vi "Teleop.vi"(1 "PreValue 2":bool, 3 "PreValue":bool, 9 "PreValue 3":bool, 10 "Match Info":T1={"Autonomous Elapsed Seconds"=0.0, "TeleOp Elapsed Seconds"=0.0, "Disabled Elapsed Seconds"=0.0, "Visited Autonomous"=FALSE, "Visited TeleOp"=FALSE, "Visited Disabled"=FALSE, "Autonomous Settings"={"Autonomous Style"=enum."Independent", "VI Refnum"=refnum}}, 11 "Call Context":T2) -> (0 "CurrentValue 2":bool, 2 "CurrentValue":bool, 8 "CurrentValue 3":bool)   [LabVIEW 2015]
doc: "This VI is called for each TeleOp packet received from the DS where the robot is not disabled. It is often used to read from the joysticks and update I/O or to update setpoints for timed control loops. It should complete and return within 20 milliseconds or it may miss DS packets."
uses:
  <vilib>/Rock Robotics/WPI/DriverStation/WPI_DriverStationDerivedRobotMode.ctl
  <vilib>/Rock Robotics/WPI/DriverStation/WPI_DriverStationMatch Info.ctl
  <vilib>/Rock Robotics/WPI/Solenoid/WPI_SolenoidValue.ctl
  <vilib>/Rock Robotics/WPI/Utilities/WPI_GetSetVariantRefNum.vi
  <vilib>/Rock Robotics/Network Tables/NT Write Boolean.vi
  <vilib>/Rock Robotics/Network Tables/NT Write Numeric Array.vi
  <vilib>/Rock Robotics/Network Tables/NT Read Boolean.vi
  <vilib>/Rock Robotics/Network Tables/NT Read Number.vi
  Robot Global Data.vi
  <vilib>/Rock Robotics/WPI/Solenoid/WPI_SolenoidSetEnum.vi
panel:
  out "Sample Slider 0":dbl(slide) scale=0.0..5.0
  out "Sample Boolean 1":bool
  out "Sample Boolean 0":bool
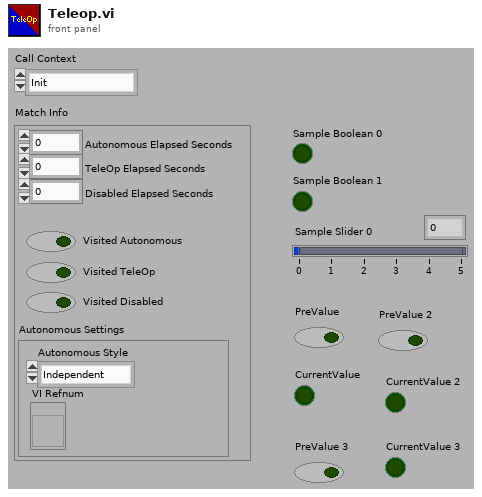
[diagram p1: front panel]
types:
  T1 = typedef "WPI_DriverStationMatch Info.ctl" = cluster{"Autonomous Elapsed Seconds":dbl, "TeleOp Elapsed Seconds":dbl, "Disabled Elapsed Seconds":dbl, "Visited Autonomous":bool, "Visited TeleOp":bool, "Visited Disabled":bool, "Autonomous Settings":cluster{"Autonomous Style":enum16{"Iterative", "Independent"}, "VI Refnum":refnum<vi>}}
  T2 = typedef "WPI_DriverStationDerivedRobotMode.ctl" = enum16{"Init", "Execute", "Stop"}
  T3 = typedef "WPI_SolenoidValue.ctl" = enum16{"Off", "On", "Forward", "Reverse"}
  T4 = typedef "WPI_RobotDriveDevRef.ctl" = cluster{"DevStatus":errorcluster, "Motors[]":T5[], "Square Inputs":bool, "Max Output":dbl}
  T5 = typedef "WPI_MotorControlDeviceRef.ctl" = cluster{"DeviceStatus":errorcluster, "Type":T6, "PWM":cluster{"PWM Channel":T7, "DeadBand":T8}, "CAN":cluster{"Device Number":u8, "Control Mode":T9, "Semaphore":T10, "Max Vout":dbl, "TalonSRX Control Mode":T11}, "Invert":bool}
  T6 = typedef "WPI_MotorControlType.ctl" = enum16{"PWM", "CAN", "CANTalonSRX"}
  T7 = typedef "FPGA_DIOPWMChannel.ctl" = enum8{"PWM 0", "PWM 1", "PWM 2", "PWM 3", "PWM 4", "PWM 5", "PWM 6", "PWM 7", "PWM 8", "PWM 9", "PWM MXP 0", "PWM MXP 1", "PWM MXP 2", "PWM MXP 3", "PWM MXP 4", "PWM MXP 5", "PWM MXP 6", "PWM MXP 7", "PWM MXP 8", "PWM MXP 9", "Invalid"}
  T8 = typedef "WPI_PWMDeadband.ctl" = cluster{"Name":string, "maxPositivePwm":i32, "minPositivePwm":i32, "centerPwm":i32, "maxNegativePwm":i32, "minNegativePwm":i32, "angularRange":u16}
  T9 = typedef "WPI_CANJaguar_ControlMode.ctl" = enum8{"Percent VBus", "Current", "Speed", "Position", "Voltage"}
  T10 = typedef "Semaphore RefNum" = refnum<k1>
  T11 = typedef "WPI_CANTalonSRX_APIControlMode.ctl" = enum8{"Percent VBus", "Speed", "Position", "Slave", "Unchanged / Invalid", "Voltage Compensation", "Current", "Motion Profile"}
  T12 = typedef "WPI_JoystickDevRef.ctl" = cluster{"Device":T13}
  T13 = typedef "WPI_JoystickDeviceEnum.ctl" = enum16{"USB 0", "USB 1", "USB 2", "USB 3", "USB 4", "USB 5"}
  T14 = cluster{"Buttons[0]":bool, "Buttons[1]":bool, "Buttons[2]":bool, "Buttons[3]":bool, "Buttons[4]":bool, "Buttons[5]":bool, "Buttons[6]":bool, "Buttons[7]":bool, "Buttons[8]":bool}
  T15 = typedef "WPI_DigitalInputDevRef.ctl" = cluster{"DevStatus":errorcluster, "DIO Channel":T16}
  T16 = typedef "FPGA_DIOChannel.ctl" = enum8{"DIO 0", "DIO 1", "DIO 2", "DIO 3", "DIO 4", "DIO 5", "DIO 6", "DIO 7", "DIO 8", "DIO 9", "DIO MXP 0", "DIO MXP 1", "DIO MXP 2", "DIO MXP 3", "DIO MXP 4", "DIO MXP 5", "DIO MXP 6", "DIO MXP 7", "DIO MXP 8", "DIO MXP 9", "DIO MXP 10", "DIO MXP 11", "DIO MXP 12", "DIO MXP 13", "DIO MXP 14", "DIO MXP 15", "Invalid"}
  T17 = typedef "WPI_SolenoidDevRef.ctl" = cluster{"DevStatus":errorcluster, "Pneumatics Control Module":u8, "Forward Solenoid Channel":T18, "Reverse Solenoid Channel":T18}
  T18 = typedef "WPI_SolenoidChannel.ctl" = enum8{"Solenoid 0", "Solenoid 1", "Solenoid 2", "Solenoid 3", "Solenoid 4", "Solenoid 5", "Solenoid 6", "Solenoid 7", "Invalid"}
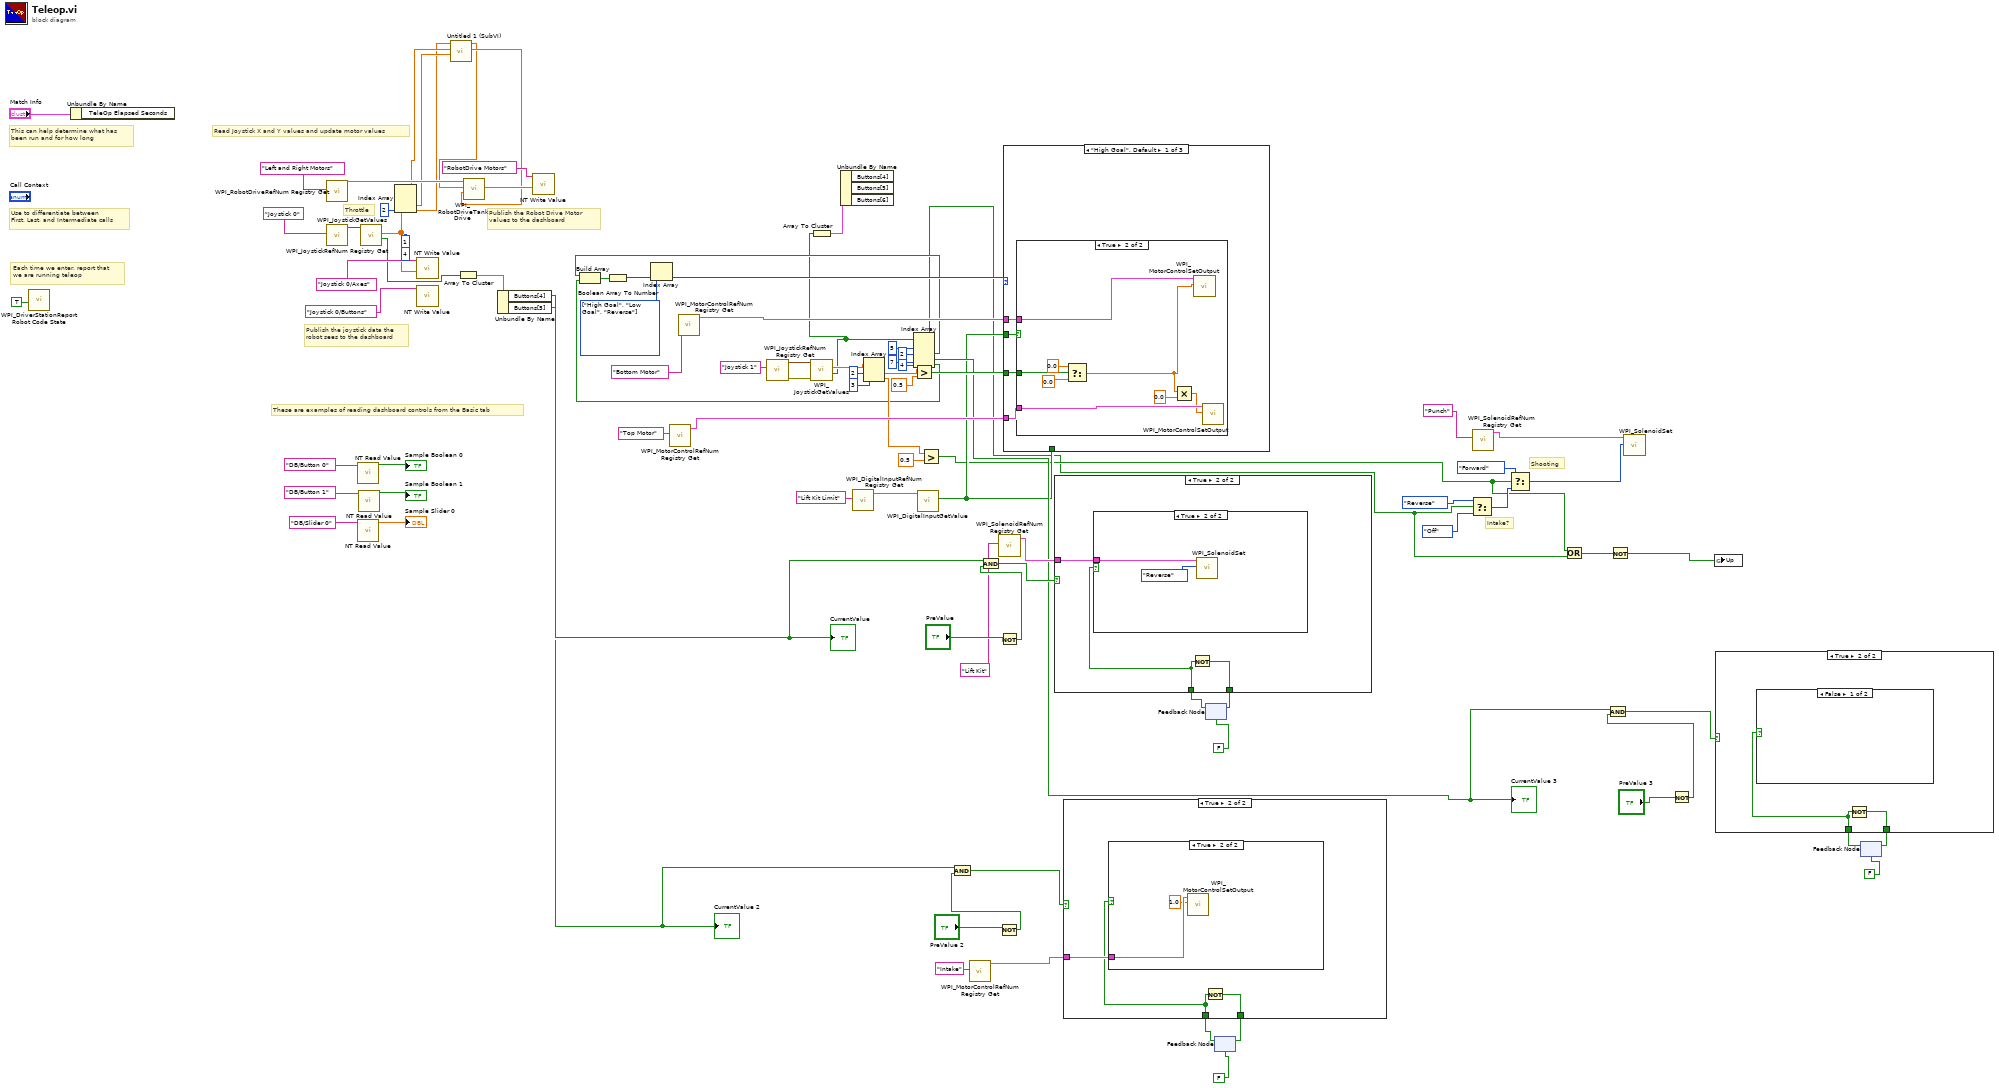
[diagram p0: block diagram]
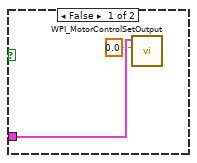
[diagram p5: hidden frame]
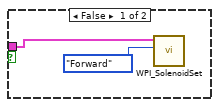
[diagram p7: hidden frame]
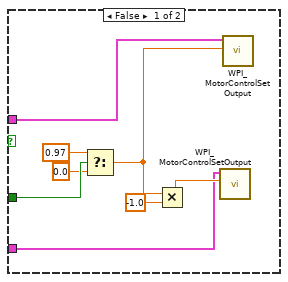
[diagram p8: hidden frame]
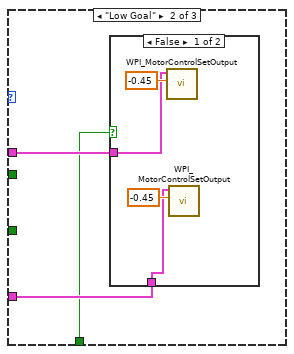
[diagram p9: hidden frame]
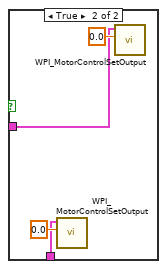
[diagram p10: hidden frame]
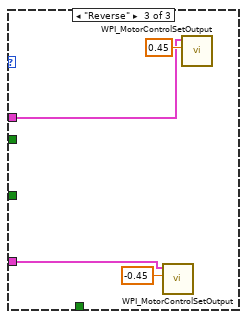
[diagram p11: hidden frame]
diagram:
  w75 = enum16{"High Goal", "Low Goal", "Reverse", ""}[] [enum."High Goal", enum."Low Goal", enum."Reverse"] items=["High Goal", "Low Goal", "Reverse", ""] ("array")
  # "Throttle"
  # "Intake?"
  # "Shooting"
  # "These are examples of reading dashboard controls from the Basic tab"
  # "Publish the Robot Drive Motor\nvalues to the dashboard"
  # "Publish the joystick data the\nrobot sees to the dashboard"
  # "Each time we enter, report that\nwe are running teleop"
  # "Use to differentiate between\nFirst, Last, and Intermediate calls"
  # "This can help determine what has\nbeen run and for how long"
  # "Read Joystick X and Y values and update motor values"
  n1 = call <vilib>:"WPI_DriverStationReport Robot Code State.vi"("TeleOp"=TRUE ("Autonomous")) -> ()  [unwired: 10 in, 1 out]
  n2 = Unbundle By Name("Match Info") -> ()  [unwired: 1 out]
  n3 = call <vilib>:"WPI_RobotDriveRefNum Registry Get.vi"("refnum name"="Left and Right Motors") -> ("RobotDriveDevRef"=w58:T4)  [unwired: 1 in, 9 out]
  n4 = call <vilib>:"WPI_JoystickRefNum Registry Get.vi"("refnum name"="Joystick 0") -> ("JoystickDevRef"=w90:T12)  [unwired: 1 in, 9 out]
  n5 = call-poly <vilib>:"NT Read Value.vi"("Name"="DB/Button 0" ("refnum name")) -> ("Boolean"=→"Sample Boolean 0":bool)  [unwired: 9 in, 1 out]
  n6 = call-poly <vilib>:"NT Read Value.vi"("Name"="DB/Slider 0" ("refnum name")) -> ("Numeric"=→"Sample Slider 0":dbl)  [unwired: 9 in, 1 out]
  n7 = call-poly <vilib>:"NT Read Value.vi"("Name"="DB/Button 1" ("refnum name")) -> ("Boolean"=→"Sample Boolean 1":bool)  [unwired: 9 in, 1 out]
  n8 = call <vilib>:"WPI_JoystickGetValues.vi"("JoystickDevRef"=w90) -> ("Buttons"=w71:bool[], "Axes"=w86:dbl[])  [unwired: 6 in, 3 out]
  n9 = Index Array(array=w86, index #1=1 ("index"), index #2=4 ("index"), index #3=2 ("index")) -> (element #1=w28:dbl, element #2=w29:dbl, element #3=w24:dbl)
  n10 = call-poly <vilib>:"NT Write Value.vi"("Numeric Array"=w86, "Name"="Joystick 0/Axes") -> ()  [unwired: 9 in, 1 out]
  n11 = call-poly <vilib>:"NT Write Value.vi"("Name"="Joystick 0/Buttons") -> ()  [unwired: 10 in, 1 out]
  n12 = call "Untitled 1 (SubVI).vi"("upper limit 2"=w29, "upper limit"=w28, "Throttle"=w24) -> ("Numeric 2"=w57:dbl, "Numeric"=w56:dbl)  [unwired: 7 in]
  n13 = Array To Cluster(array=w71) -> (cluster=w78:T14)
  n14 = call <vilib>:"WPI_RobotDriveTankDrive.vi"("Right axis value"=w57, "Left axis value"=w56, "RobotDriveDevRef"=w58) -> ("Motor Values"=w59:dbl[])  [unwired: 6 in, 2 out]
  n15 = Unbundle By Name(w78) -> ("Buttons[4]"=w68:bool, "Buttons[5]"=w32:bool)
  "CurrentValue" <- w68
  "CurrentValue 2" <- w32
  n16 = call-poly <vilib>:"NT Write Value.vi"("Numeric Array"=w59, "Name"="RobotDrive Motors") -> ()  [unwired: 9 in, 1 out]
  n17 = call <vilib>:"WPI_MotorControlRefNum Registry Get.vi"("refnum name"="Top Motor") -> ("MotorControlDevRef"=w69:T5)  [unwired: 9 in, 1 out]
  n18 = call <vilib>:"WPI_MotorControlRefNum Registry Get.vi"("refnum name"="Bottom Motor") -> ("MotorControlDevRef"=w73:T5)  [unwired: 9 in, 1 out]
  n19 = call <vilib>:"WPI_JoystickRefNum Registry Get.vi"("refnum name"="Joystick 1") -> ("error out"=w52:errorcluster, "JoystickDevRef"=w51:T12)  [unwired: 1 in, 8 out]
  n20 = call <vilib>:"WPI_JoystickGetValues.vi"("error in (no error)"=w52, "JoystickDevRef"=w51) -> ("Buttons"=w2:bool[], "Axes"=w49:dbl[])  [unwired: 5 in, 3 out]
  n21 = Array To Cluster(array=w2) -> (cluster=w1:T14)
  n22 = Unbundle By Name(w1) -> ()  [unwired: 3 out]
  n23 = call <vilib>:"WPI_DigitalInputRefNum Registry Get.vi"("refnum name"="Lift Kit Limit") -> ("DigitalInputDevRef"=w9:T15)  [unwired: 9 in, 1 out]
  n24 = Index Array(array=w49, index #1=2 ("index"), index #2=3 ("index")) -> (element #1=w48:dbl, element #2=w43:dbl)
  n25 = Index Array(array=w2, index #1=5 ("index"), index #2=2 ("index"), index #3=7 ("index"), index #4=4 ("index")) -> (element #1=w5:bool, element #2=w12:bool, element #3=w18:bool, element #4=w10:bool)
  "CurrentValue 3" <- w18
  n26 = Build Array(w12, w10) -> (w77:bool[])
  n27 = Boolean Array To Number(Boolean array=w77) -> (number=w76:u32)
  n28 = Index Array(array=w75, index=w76) -> (element=w74:enum16{"High Goal", "Low Goal", "Reverse", ""})
  n29 = Greater?(x=w48, y=0.5) -> (0:w46:bool)
  n30 = call <vilib>:"WPI_DigitalInputGetValue.vi"("DigitalInputDevRef"=w9) -> ("Value"=w7:bool)  [unwired: 8 in, 2 out]
  n31 = Greater?(x=w43, y=0.5) -> (0:w6:bool)
  n32 = call <vilib>:"WPI_MotorControlRefNum Registry Get.vi"("refnum name"="Intake") -> ("MotorControlDevRef"=w34:T5)  [unwired: 9 in, 1 out]
  n33 = Not(x="PreValue 2") -> (.not. x?=w31:bool)
  n34 = And(x=w32, y=w31) -> (x .and. y?=w30:bool)
  n35 = call <vilib>:"WPI_SolenoidRefNum Registry Get.vi"("refnum name"="Lift Kit") -> ("SolenoidDevRef"=w60:T17)  [unwired: 9 in, 1 out]
  n36 = Not(x="PreValue") -> (.not. x?=w66:bool)
  n37 = And(x=w68, y=w66) -> (x .and. y?=w65:bool)
  n38 = case shown="\"High Goal\", Default" w74 {
    tunnel: w73 -> [w97 w116 w127]
    tunnel: w69 -> [w96 w115 w125]
    tunnel: w46 -> [w95 _ _]
    tunnel: w7 -> [_ w114 _]
    tunnel: w7 -> [w94 _ _]
    frame "High Goal", Default {
      n39 = case shown="True" w94 {
        tunnel: w97 -> [w99 w113]
        tunnel: w96 -> [w98 w112]
        tunnel: w95 -> [w104 w111]
        frame False {
          n40 = Select(t=0.97, s=w104, f=0.0) -> (s? t:f=w103:dbl)
          n41 = Multiply(x=w103, y=-1.0) -> (x*y=w105:dbl)
          n42 = call <vilib>:"WPI_MotorControlSetOutput.vi"("Output"=w105, "MotorControlDevRef"=w98) -> ()  [unwired: 7 in, 3 out]
          n43 = call <vilib>:"WPI_MotorControlSetOutput.vi"("Output"=w103, "MotorControlDevRef"=w99) -> ()  [unwired: 7 in, 3 out]
        }
        frame True {
          n44 = Select(t=0.0, s=w111, f=0.0) -> (s? t:f=w109:dbl)
          n45 = Multiply(x=w109, y=0.0) -> (x*y=w107:dbl)
          n46 = call <vilib>:"WPI_MotorControlSetOutput.vi"("Output"=w109, "MotorControlDevRef"=w113) -> ()  [unwired: 7 in, 3 out]
          n47 = call <vilib>:"WPI_MotorControlSetOutput.vi"("Output"=w107, "MotorControlDevRef"=w112) -> ()  [unwired: 7 in, 3 out]
        }
      }
    }
    frame "Low Goal" {
      n48 = case shown="False" w114 {
        tunnel: w116 -> [w117 w123]
        tunnel: w115 -> [w118 w121]
        frame False {
          n49 = call <vilib>:"WPI_MotorControlSetOutput.vi"("Output"=-0.45, "MotorControlDevRef"=w117) -> ()  [unwired: 7 in, 3 out]
          n50 = call <vilib>:"WPI_MotorControlSetOutput.vi"("Output"=-0.45, "MotorControlDevRef"=w118) -> ()  [unwired: 7 in, 3 out]
        }
        frame True {
          n51 = call <vilib>:"WPI_MotorControlSetOutput.vi"("Output"=0.0, "MotorControlDevRef"=w121) -> ()  [unwired: 7 in, 3 out]
          n52 = call <vilib>:"WPI_MotorControlSetOutput.vi"("Output"=0.0, "MotorControlDevRef"=w123) -> ()  [unwired: 7 in, 3 out]
        }
      }
    }
    frame "Reverse" {
      n53 = call <vilib>:"WPI_MotorControlSetOutput.vi"("Output"=-0.45, "MotorControlDevRef"=w125) -> ()  [unwired: 7 in, 3 out]
      n54 = call <vilib>:"WPI_MotorControlSetOutput.vi"("Output"=0.45, "MotorControlDevRef"=w127) -> ()  [unwired: 7 in, 3 out]
    }
  }
  n55 = feedback #1(FALSE) -> (w62:bool)
  n56 = case shown="True" w65 {
    tunnel: [w129 w132] -> w63
    tunnel: w62 -> [w129 w130]
    tunnel: w60 -> [_ w131]
    frame False {
    }
    frame True {
      n57 = case shown="True" w130 {
        tunnel: w131 -> [w134 w136]
        frame False {
          n58 = call-poly <vilib>:"WPI_SolenoidSet.vi"("Value"=WPI_SolenoidValue."Forward", "SolenoidDevRef"=w134) -> ()  [unwired: 8 in, 2 out]
        }
        frame True {
          n59 = call-poly <vilib>:"WPI_SolenoidSet.vi"("Value"=WPI_SolenoidValue."Reverse", "SolenoidDevRef"=w136) -> ()  [unwired: 8 in, 2 out]
        }
      }
      n60 = Not(x=w130) -> (.not. x?=w132:bool)
    }
  }
  n61 = feedback-in #1(w63) -> ()
  n62 = feedback #2(FALSE) -> (w35:bool)
  n63 = case shown="True" w30 {
    tunnel: [w137 w140] -> w36
    tunnel: w35 -> [w137 w138]
    tunnel: w34 -> [_ w139]
    frame False {
    }
    frame True {
      n64 = case shown="True" w138 {
        tunnel: w139 -> [w142 w144]
        frame False {
          n65 = call <vilib>:"WPI_MotorControlSetOutput.vi"("Output"=0.0, "MotorControlDevRef"=w142) -> ()  [unwired: 7 in, 3 out]
        }
        frame True {
          n66 = call <vilib>:"WPI_MotorControlSetOutput.vi"("Output"=1.0, "MotorControlDevRef"=w144) -> ()  [unwired: 7 in, 3 out]
        }
      }
      n67 = Not(x=w138) -> (.not. x?=w140:bool)
    }
  }
  n68 = feedback-in #2(w36) -> ()
  n69 = Select(t=WPI_SolenoidValue."Reverse" ("Value"), s=w5, f=WPI_SolenoidValue."Off" ("Value")) -> (s? t:f=w27:T3)
  n70 = call <vilib>:"WPI_SolenoidRefNum Registry Get.vi"("refnum name"="Punch") -> ("SolenoidDevRef"=w42:T17)  [unwired: 9 in, 1 out]
  n71 = Select(t=WPI_SolenoidValue."Forward" ("Value"), s=w6, f=w27) -> (s? t:f=w41:T3)
  n72 = Or(x=w6, y=w5) -> (x .or. y?=w4:bool)
  n73 = Not(x=w4) -> (.not. x?=w3:bool)
  n74 = call-poly <vilib>:"WPI_SolenoidSet.vi"("Value"=w41, "SolenoidDevRef"=w42) -> ()  [unwired: 8 in, 2 out]
  n75 = Not(x="PreValue 3") -> (.not. x?=w19:bool)
  n76 = And(x=w18, y=w19) -> (x .and. y?=w17:bool)
  n77 = global write "Robot Global Data.vi" "Up"(w3) -> ()
  n78 = feedback #3(FALSE) -> (w14:bool)
  n79 = case shown="True" w17 {
    tunnel: [w145 w147] -> w15
    tunnel: w14 -> [w145 w146]
    frame False {
    }
    frame True {
      n80 = case shown="False" w146 {
        frame False {
        }
        frame True {
        }
      }
      n81 = Not(x=w146) -> (.not. x?=w147:bool)
    }
  }
  n82 = feedback-in #3(w15) -> ()
